vi "tasks.vi"() -> ()   [LabVIEW 2013]
panel:
  out "tasks":T1
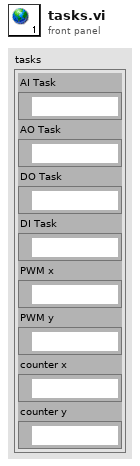
[diagram p1: front panel]
types:
  T1 = cluster{"AI Task":refnum<k21>, "AO Task":refnum<k21>, "DO Task":refnum<k21>, "DI Task":refnum<k21>, "PWM x":refnum<k21>, "PWM y":refnum<k21>, "counter x":refnum<k21>, "counter y":refnum<k21>}
diagram:
